vi "Read Finish On.vi"(8 "error in (no error)":errorcluster, 11 "Repeater in":refnum<class "Repeater.lvclass">) -> (0 "error out":errorcluster, 2 "Finish On":T1, 3 "Repeater out":refnum<class "Repeater.lvclass">)   [LabVIEW 2021, in "BT.lvlib" / "Repeater.lvclass"]
uses:
  Repeater.lvclass
  Support/Finish On - Type.ctl
  Repeater.lvclass/Repeater.ctl
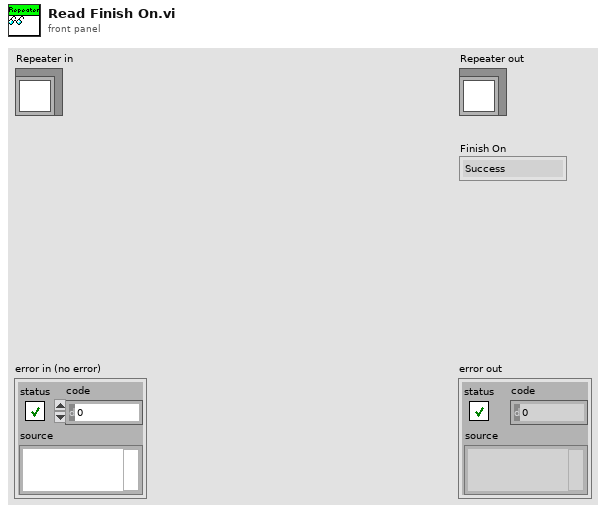
[diagram p1: front panel]
types:
  T1 = typedef "BT.lvlib/Repeater.lvclass/Finish On - Type.ctl" = enum16{"Success", "Failure", "Never"}
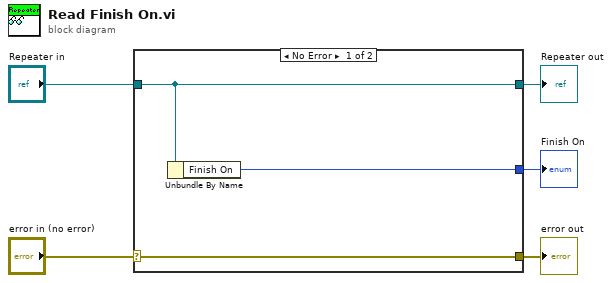
[diagram p0: block diagram]
diagram:
  n1 = case shown="No Error" "error in (no error)" {
    selector: "error in (no error)" -> [w8 w9]
    tunnel: [w8 w9] -> w4
    tunnel: [w7 w10] -> w2
    tunnel: "Repeater in" -> [w7 w10]
    tunnel: [w6 _] -> w1
    frame No Error {
      n2 = Unbundle By Name(w7) -> ("Finish On"=w6:T1)
    }
    frame Error {
    }
  }
  "error out" <- w4
  "Repeater out" <- w2
  "Finish On" <- w1
